vi "4.BalancingTest.vi"() -> ()   [LabVIEW 2019, in "SJCube_KNRm.lvlib"]
uses:
  SJCube_KNRm.lvlib
  <vilib>/Platform/TimedLoop/XDataNode/timing_clust.ctl
  <vilib>/Platform/TimedLoop/XDataNode/nitl_modes.ctl
  <vilib>/Platform/TimedLoop/XDataNode/wakeup.ctl
  KNRm_ReMi_OS5.lvlibp/KNRm_ReMi_Toolkit/IO/LowLevel/IO_Channel_DIO.ctl
  <vilib>/addons/control/pid/pid.llb/PID (DBL).vi
  <vilib>/Platform/TimedLoop/XDataNode/XDataNode.xnode
  <vilib>/addons/control/pid/NI_PID_pid.lvlib
  <vilib>/Platform/TimedLoop/XDataNode/XDNodeRunTimeDep.lvlib
  KNRm_ReMi_OS5.lvlibp
panel:
  out "output":dbl format="%.2f"
  out "x-y":dbl
  out "Err":dbl
  out "Waveform Chart":T1(graph)
  in  "star":bool
  in  "Stop Button":bool
  in  "Reset":bool
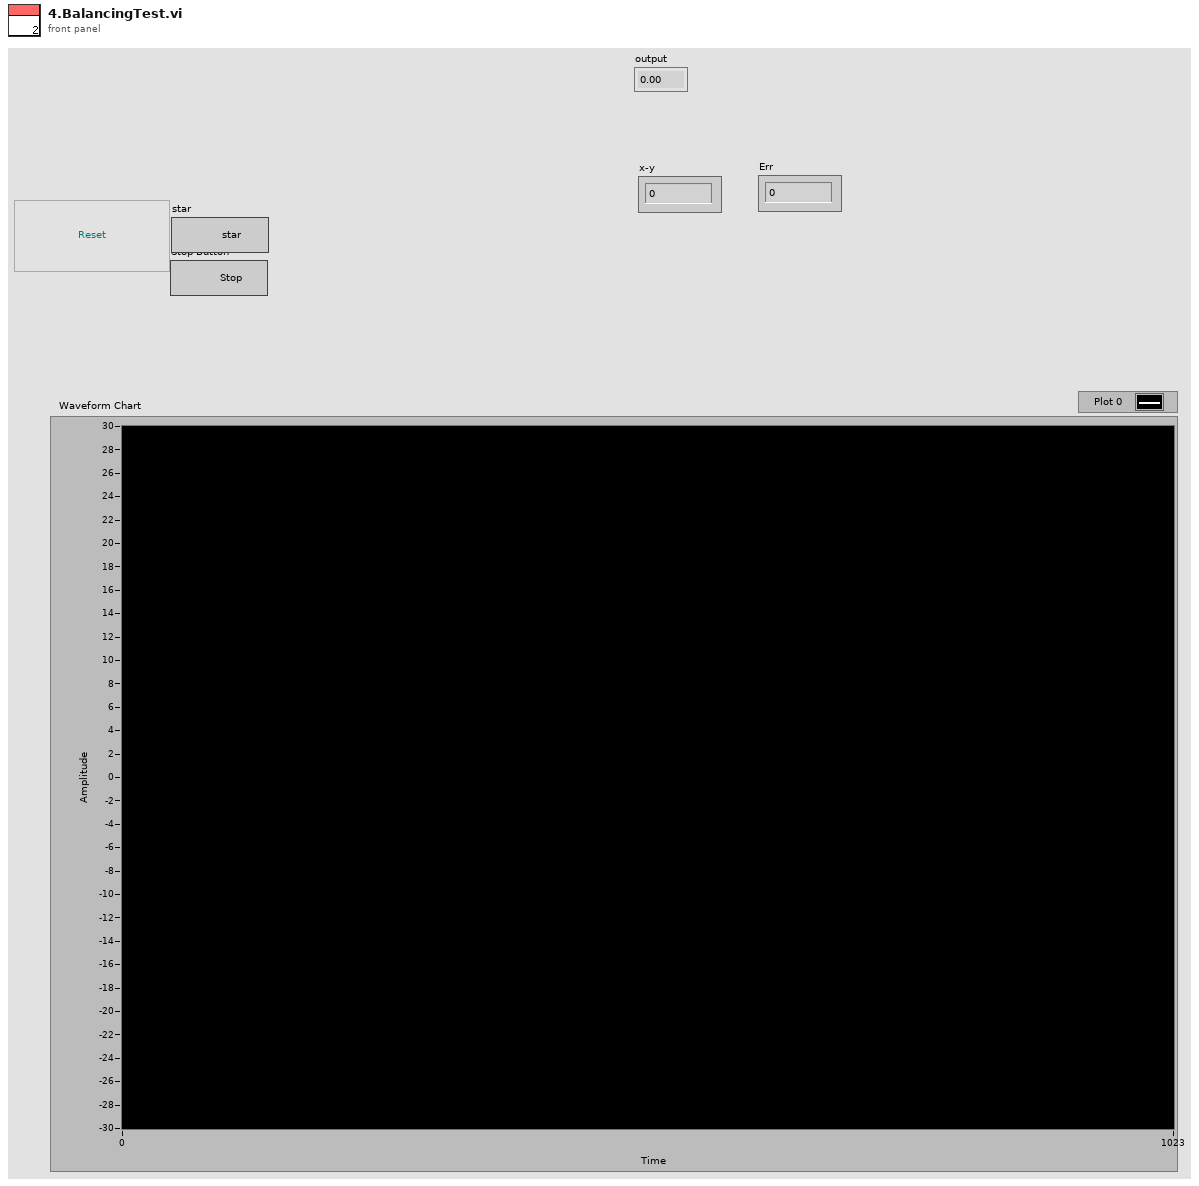
[diagram p1: front panel]
types:
  T1 = cluster{"Position (deg)":dbl, "MotorEncoder (deg)":dbl}
  T2 = typedef "KNRm_ReMi_OS5.lvlibp/IO_Channel_DIO.ctl" = enum16{"B/DIO1 (M1)", "A/DIO8 (M2)", "B/DIO7 (M3)", "A/DIO3 (M4)", "A/DIO14 (RC1_0)", "A/DIO15 (RC1_1)"}
  T3 = typedef "XDNodeRunTimeDep.lvlib/timing_clust.ctl" = cluster{"Expected End [f-1]":u64, "Actual End [f-1]":u64, "Finished Late? [f-1]":bool, "Expected End [i-1]":u64, "Actual End [i-1]":u64, "Finished Late? [i-1]":bool, "Expected Start [i]":u64, "Actual Start [i]":u64, "Expected Start [f]":u64, "Actual Start [f]":u64, "Source Name":string, "Structure Name":string, "Period":i64, "Deadline":i64, "Offset":i64, "Start":i64, "Priority":i32, "Timeout":i32, "Mode":T4, "Wakeup Reason":T5, "Error":errorcluster, "Source Type":string, "Secondary Source Type":string, "Global End Time":u64, "Global Start Time":u64, "Frame Duration":u64, "Iteration Duration":u64, "Assigned CPU":i32, "I/O Scan Engine Mode":u32}
  T4 = typedef "XDNodeRunTimeDep.lvlib/nitl_modes.ctl" = enum32{"No Change", "Process missed periods, maintain original phase", "Discard missed periods, maintain original phase", "Process missed periods, ignore original phase", "Discard missed periods, ignore original phase"}
  T5 = typedef "XDNodeRunTimeDep.lvlib/wakeup.ctl" = enum32{"Normal", "Aborted", "Asynchronous wakeup", "Timing source error", "Timed loop error", "Timeout"}
  T6 = cluster{"proportional gain (Kc)":dbl, "integral time (Ti, min)":dbl, "derivative time (Td, min)":dbl}
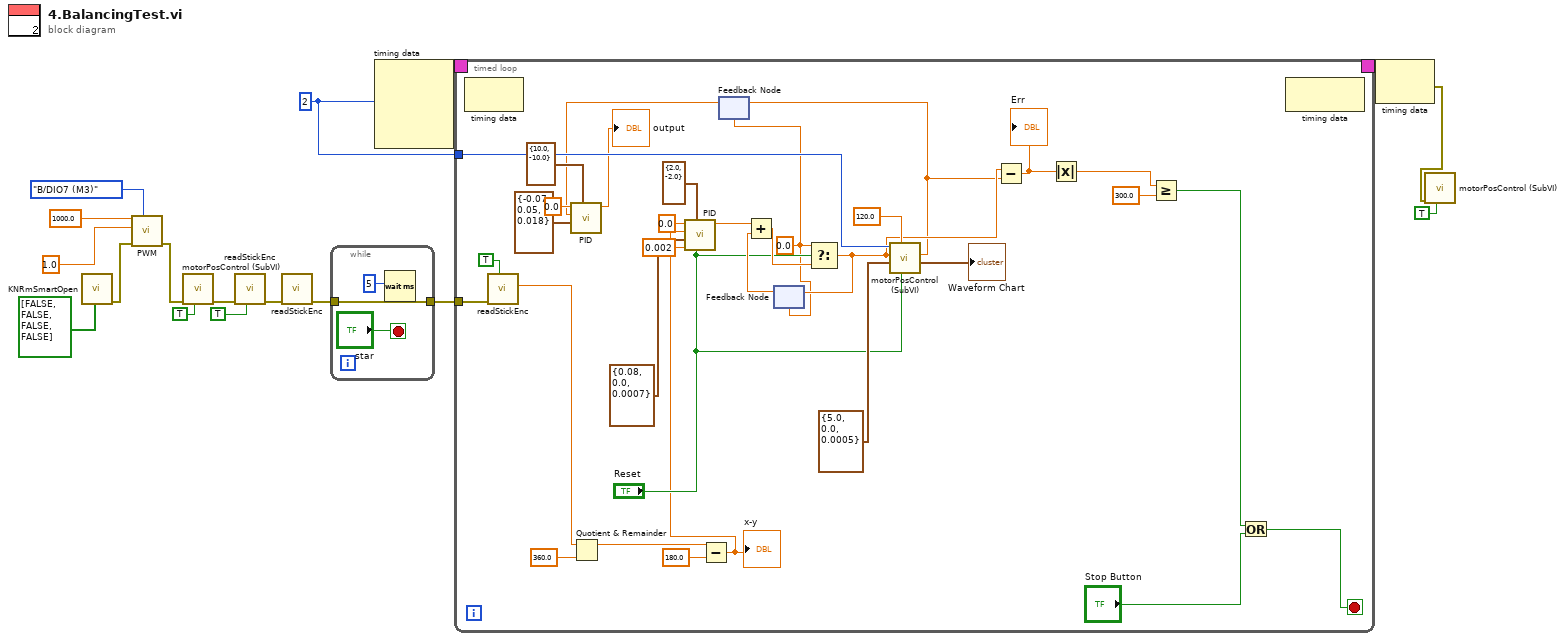
[diagram p0: block diagram]
diagram:
  w15 = i64 2 ("Period")
  n1 = call "KNRmSmartOpen.vi"("SpeedMode"=bool[] [FALSE, FALSE, FALSE, FALSE]) -> ("error out"=w2:errorcluster)  [unwired: 8 in, 2 out]
  n2 = call "PWM.vi"("IO_Chanel"=IO_Channel_DIO."B/DIO7 (M3)", "error in"=w2, "DutyCycle"=1.0, "Frequency(Hz)"=1000.0) -> ("error out"=w1:errorcluster)  [unwired: 7 in]
  n3 = call "motorPosControl (SubVI).vi"("Reset"=TRUE, "error in (no error)"=w1) -> ("error out"=w12:errorcluster)  [unwired: 6 in, 3 out]
  n4 = call "readStickEnc.vi"("Reset Counter"=TRUE, "error in (no error)"=w12) -> ("error out"=w8:errorcluster)  [unwired: 8 in, 1 out]
  n5 = call "readStickEnc.vi"("error in (no error)"=w8) -> ("error out"=w7:errorcluster)  [unwired: 9 in, 1 out]
  n6 = while {
    tunnel: w7 -> [w20]
    tunnel: [w20] -> w13
    stop <- "star" stop-if-true
    n7 = Wait (ms)(milliseconds to wait=u32 5) -> ()  [unwired: 1 out]
  }
  n8 = node-c288(w15) -> (w17:T3)  [unwired: 3 in]
  n9 = timed-loop {
    timing: w17 -> [_]
    timing-out: [_] -> w16
    tunnel: w15 -> [w46]
    tunnel: w13 -> [w44]
    stop <- w36 stop-if-true
    w23 = 0.0 ("t")
    n10 = node-c288() -> ()  [unwired: 1 in, 1 out]
    n11 = call "readStickEnc.vi"("Reverse ENC?"=TRUE, "error in (no error)"=w44) -> ("StickEncoder (deg)"=w41:dbl)  [unwired: 8 in, 1 out]
    n12 = Quotient & Remainder(x=w41, y=360.0) -> (x-y*floor(x/y)=w40:dbl)  [unwired: 1 out]
    n13 = Subtract(x=w40, y=180.0) -> (x-y=w29:dbl)
    "x-y" <- w29
    n14 = call-poly <vilib>:"PID.vi"("reinitialize? (F)"="Reset", "output range"=cluster{"output high":dbl, "output low":dbl} {"output high"=2.0, "output low"=-2.0}, "dt (s)"=0.002, "PID gains"=T6 {"proportional gain (Kc)"=0.08, "integral time (Ti, min)"=0.0, "derivative time (Td, min)"=0.0007}, "process variable"=w29, "setpoint"=0.0) -> ("output"=w52:dbl)  [unwired: 4 in, 1 out]
    n15 = feedback #1(w23) -> (w25:dbl)
    n16 = call-poly <vilib>:"PID.vi"("output range"=cluster{"output high":dbl, "output low":dbl} {"output high"=10.0, "output low"=-10.0}, "PID gains"=T6 {"proportional gain (Kc)"=-0.07, "integral time (Ti, min)"=0.05, "derivative time (Td, min)"=0.018}, "process variable"=w25, "setpoint"=0.0) -> ("output"=→"output":dbl)  [unwired: 6 in, 1 out]
    n17 = feedback #2(w23) -> (w51:dbl)
    n18 = Add(x=w52, y=w51) -> (x+y=w50:dbl)
    n19 = Select(t=w23, s="Reset", f=w50) -> (s? t:f=w35:dbl)
    n20 = feedback-in #2(w35) -> ()
    n21 = call "motorPosControl (SubVI).vi"("Reset"="Reset", "+/- Range"=120.0, "PID gains"=T6 {"proportional gain (Kc)"=5.0, "integral time (Ti, min)"=0.0, "derivative time (Td, min)"=0.0005}, "Position (deg)"=w35, "dt"=w46) -> ("Waveform Chart"=→"Waveform Chart":T1, "MotorEncoder (deg)"=w24:dbl)  [unwired: 3 in, 2 out]
    n22 = feedback-in #1(w24) -> ()
    n23 = Subtract(x=w35, y=w24) -> (x-y=w32:dbl)
    "Err" <- w32
    n24 = Absolute Value(x=w32) -> (abs(x)=w31:dbl)
    n25 = Greater Or Equal?(x=w31, y=300.0) -> (x >= y?=w33:bool)
    n26 = Or(x=w33, y="Stop Button") -> (x .or. y?=w36:bool)
    n27 = node-c288() -> ()  [unwired: 1 in, 1 out]
  }
  n28 = node-c288(w16) -> (w9:errorcluster)
  n29 = call "motorPosControl (SubVI).vi"("Reset"=TRUE, "error in (no error)"=w9) -> ()  [unwired: 6 in, 4 out]
